vi "Read Joysticks.vi"() -> (0 "Manipulator Axes":T1, 1 "Manipulator Buttons":T2, 2 "Driver Axes":T1, 3 "Driver Buttons":T2)   [LabVIEW 2013]
uses:
  <vilib>/Rock Robotics/WPI/Joystick/WPI_JoystickButtonState.ctl
  <vilib>/Rock Robotics/WPI/Joystick/WPI_JoystickGetSetRefNum.vi
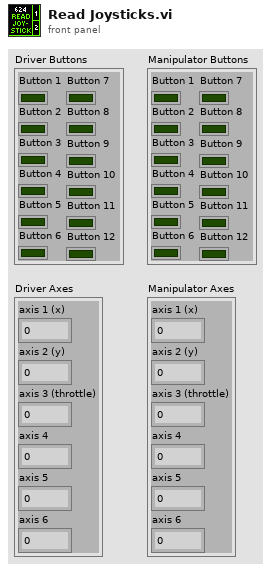
[diagram p1: front panel]
types:
  T1 = cluster{"axis 1 (x)":dbl, "axis 2 (y)":dbl, "axis 3 (throttle)":dbl, "axis 4":dbl, "axis 5":dbl, "axis 6":dbl}
  T2 = typedef "WPI_JoystickButtonState.ctl" = cluster{"Button 1":bool, "Button 2":bool, "Button 3":bool, "Button 4":bool, "Button 5":bool, "Button 6":bool, "Button 7":bool, "Button 8":bool, "Button 9":bool, "Button 10":bool, "Button 11":bool, "Button 12":bool}
  T3 = typedef "WPI_JoystickDevRef.ctl" = cluster{"Device":T4}
  T4 = typedef "WPI_JoystickDeviceEnum.ctl" = enum16{"USB 1", "USB 2", "USB 3", "USB 4", "Kinect 1", "Kinect 2"}
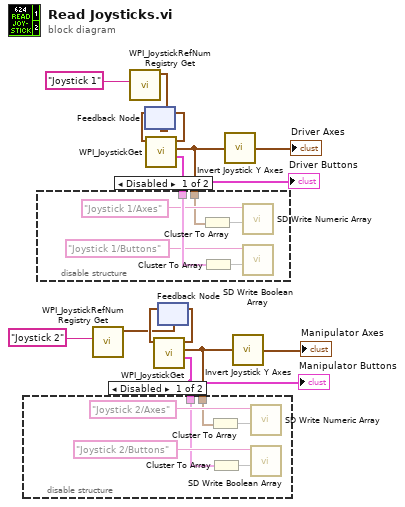
[diagram p0: block diagram]
diagram:
  n1 = call <vilib>:"WPI_JoystickRefNum Registry Get.vi"("refnum name"="Joystick 2") -> ("JoystickDevRef"=w5:T3)  [unwired: 1 in, 9 out]
  n2 = call <vilib>:"WPI_JoystickRefNum Registry Get.vi"("refnum name"="Joystick 1") -> ("JoystickDevRef"=w8:T3)  [unwired: 1 in, 9 out]
  n3 = feedback #1(w8) -> (w9:T3)
  n4 = call <vilib>:"WPI_JoystickGet.vi"("JoystickDevRef"=w9) -> ("Buttons"=w14:T2, "Axes"=w3:T1, "JoystickDevRef"=w10:T3)  [unwired: 1 in, 3 out]
  "Driver Buttons" <- w14
  n5 = disable-structure shown="Disabled" {
    disable-tunnel: w14 -> [w20 _]
    disable-tunnel: w3 -> [w17 _]
    frame Disabled {
      n6 = Cluster To Array(cluster=w17) -> (array=w18:dbl[])
      n7 = Cluster To Array(cluster=w20) -> (array=w15:bool[])
      n8 = call <vilib>:"SD Write Numeric Array.vi"("Numeric Array"=w18, "Name"="Joystick 1/Axes") -> ()  [unwired: 8 in, 2 out]
      n9 = call <vilib>:"SD Write Boolean Array.vi"("Boolean Array"=w15, "Name"="Joystick 1/Buttons") -> ()  [unwired: 8 in, 2 out]
    }
    frame Enabled {
    }
  }
  n10 = feedback-in #1(w10) -> ()
  n11 = feedback #2(w5) -> (w6:T3)
  n12 = call <vilib>:"WPI_JoystickGet.vi"("JoystickDevRef"=w6) -> ("Buttons"=w11:T2, "Axes"=w4:T1, "JoystickDevRef"=w7:T3)  [unwired: 1 in, 3 out]
  "Manipulator Buttons" <- w11
  n13 = disable-structure shown="Disabled" {
    disable-tunnel: w4 -> [w22 _]
    disable-tunnel: w11 -> [w21 _]
    frame Disabled {
      n14 = Cluster To Array(cluster=w22) -> (array=w24:dbl[])
      n15 = Cluster To Array(cluster=w21) -> (array=w26:bool[])
      n16 = call <vilib>:"SD Write Numeric Array.vi"("Numeric Array"=w24, "Name"="Joystick 2/Axes") -> ()  [unwired: 8 in, 2 out]
      n17 = call <vilib>:"SD Write Boolean Array.vi"("Boolean Array"=w26, "Name"="Joystick 2/Buttons") -> ()  [unwired: 8 in, 2 out]
    }
    frame Enabled {
    }
  }
  n18 = feedback-in #2(w7) -> ()
  n19 = call "Invert Joystick Y Axes.vi"("Axes in"=w3) -> ("Axes out"=→"Driver Axes":T1)
  n20 = call "Invert Joystick Y Axes.vi"("Axes in"=w4) -> ("Axes out"=→"Manipulator Axes":T1)
